vi "Library Format Word List.vi"(4 "words":string[](array[string]), 5 "quote?":bool) -> (1 "formatted list":string)   [LabVIEW 2012]
doc: "Takes an array of words and formats them into a string suitable to be part of a syntactically valid english sentence."
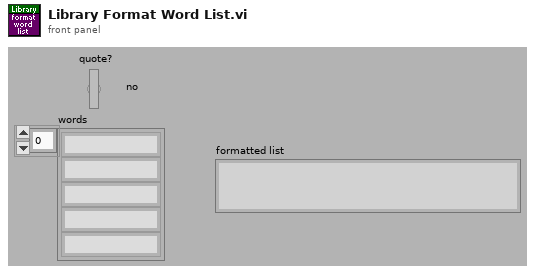
[diagram p1: front panel]
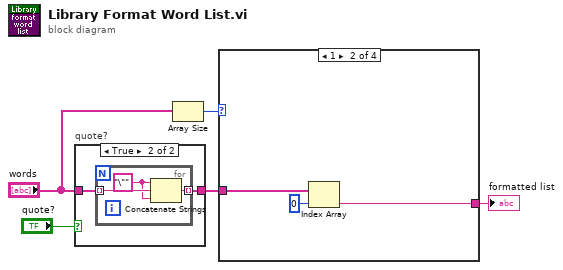
[diagram p0: block diagram]
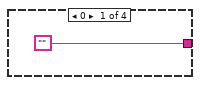
[diagram p3: hidden frame]
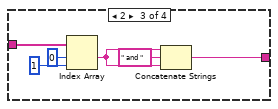
[diagram p4: hidden frame]
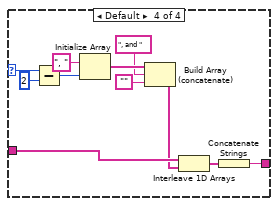
[diagram p5: hidden frame]
diagram:
  n1 = case "quote?" shown="True" "quote?" {
    tunnel: "words" -> [w6 w8]
    tunnel: [w6 w7] -> w2
    frame False {
    }
    frame True {
      n2 = for {
        tunnel: w8 -> [w11] mode=indexing
        tunnel: [w10] -> w7 mode=indexing
        w9 = "\"" ("Substring")
        n3 = Concatenate Strings(w9, w11, w9) -> (w10:string)
      }
    }
  }
  n4 = Array Size(array="words") -> (size(s)=w5:i32)
  n5 = case shown="1" w5 {
    selector: w5 -> [_ _ _ w32]
    tunnel: w2 -> [_ w15 w21 w25]
    tunnel: ["" w13 w16 w22] -> w4
    frame 0 {
    }
    frame 1 {
      n6 = Index Array(array=w15, index=0 ("Index")) -> (element=w13:string)
    }
    frame 2 {
      n7 = Index Array(array=w21, index #1=0 ("Index"), index #2=1 ("Index")) -> (element #1=w18:string)  [unwired: 1 out]
      n8 = Concatenate Strings(w18, " and " ("Substring"), w18) -> (w16:string)
    }
    frame Default {
      n9 = Subtract(x=w32, y=2) -> (x-y=w30:i32)
      n10 = Initialize Array(", ", w30) -> (w28:string[])
      n11 = Build Array (concatenate)(w28, ", and ", "") -> (w24:string[])
      n12 = Interleave 1D Arrays(w25, w24) -> (w23:string[])
      n13 = Concatenate Strings(w23) -> (w22:string)
    }
  }
  "formatted list" <- w4
